vi "tare.vi"(7 "Tare Control":bool, 9 "Shift Registor":dbl, 10 "Input Waveform":waveform(dbl)) -> (1 "Shift Registor Out":dbl, 2 "output waveform":waveform(dbl))   [LabVIEW 2018]
uses:
  <vilib>/Analysis/baseanly.llb/Mean (DBL).vi
  <vilib>/Analysis/NI_AALBase.lvlib
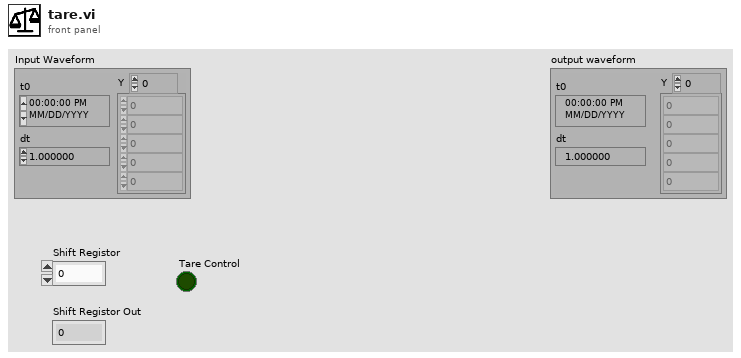
[diagram p1: front panel]
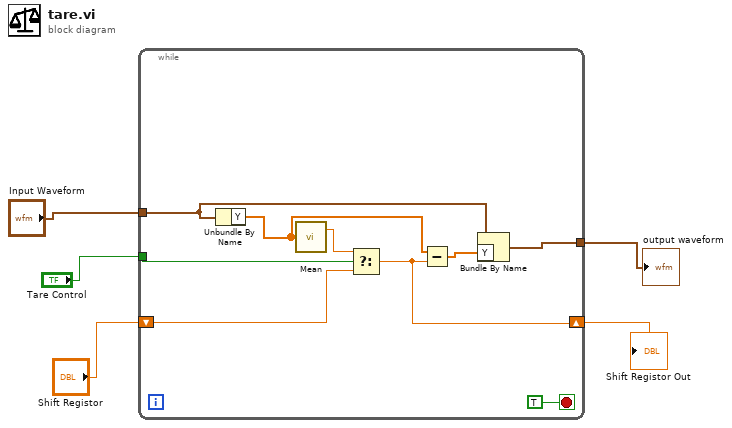
[diagram p0: block diagram]
diagram:
  n1 = while {
    tunnel: "Tare Control" -> [w11]
    tunnel: [w10] -> w4
    tunnel: "Input Waveform" -> [w8]
    shift-right: [w6] -> w1
    shift-left: "Shift Registor" -> [w7]
    stop <- TRUE stop-if-true
    n2 = Unbundle By Name(w8) -> ("Y"=w9:dbl[])
    n3 = call-poly <vilib>:"Mean.vi"("X"=w9) -> ("mean"=w13:dbl)  [unwired: 1 out]
    n4 = Select(t=w13, s=w11, f=w7) -> (s? t:f=w6:dbl)
    n5 = Subtract(x=w9, y=w6) -> (x-y=w12:dbl[])
    n6 = Bundle By Name(cluster=w8, "Y"=w12) -> (w10:waveform(dbl))
  }
  "output waveform" <- w4
  "Shift Registor Out" <- w1
